vi "initializePIP.vi"(8 "error in (no error)":errorcluster) -> (0 "error out":errorcluster, 2 "Initialize Test":string, 3 "Config and Fixture Setup":string)   [LabVIEW 2018]
uses:
  Global_1259.vi
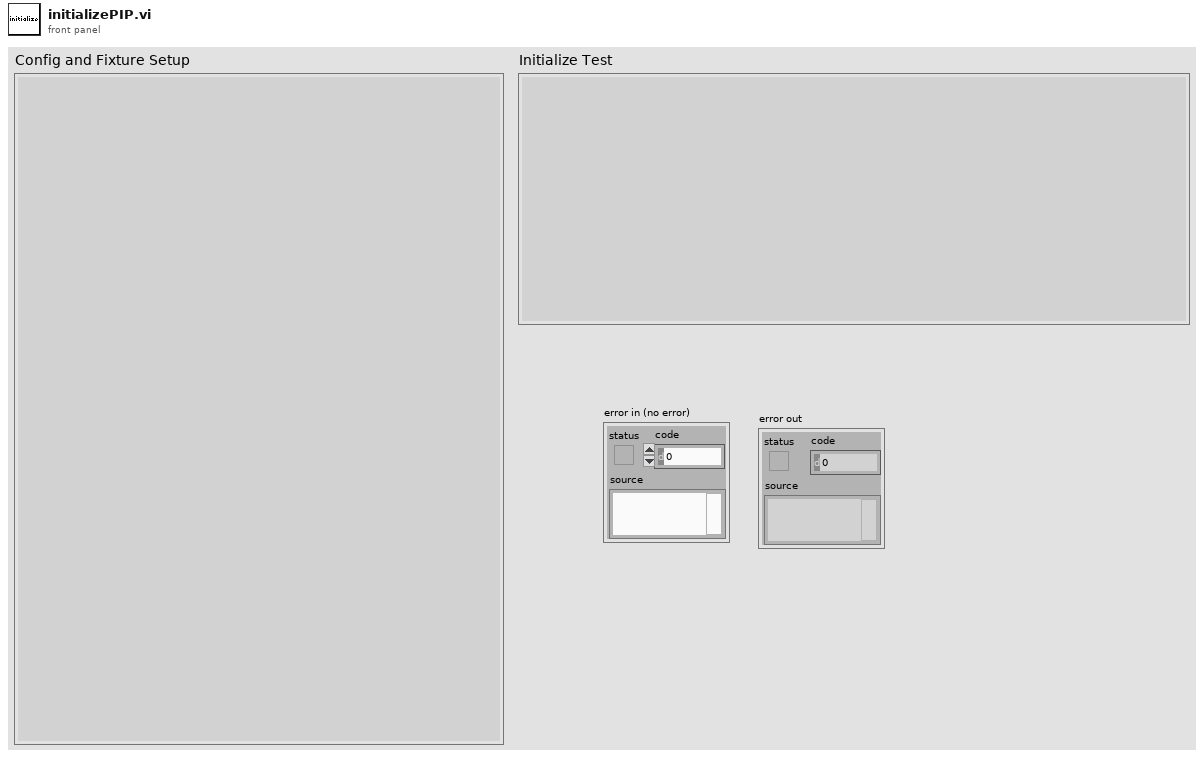
[diagram p1: front panel]
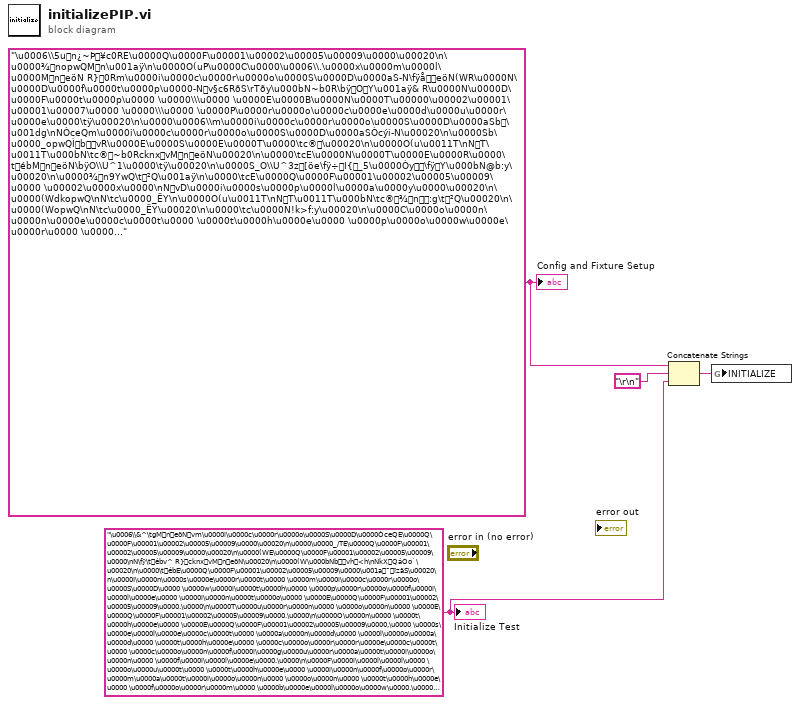
[diagram p0: block diagram]
diagram:
  w4 = "\u0006\\5un¿~Þ¥c0RE\u0000Q\u0000F\u00001\u00002\u00005\u00009\u0000\u00020\n\u0000¾nopwQMn\u001aÿ\n\u0000O(uP\u0000C\u0000\u0006\\.\u0000x\u0000m\u0000l\u0000MneöN R}0Rm\u0000i\u0000c\u0000r\u0000o\u0000S\u0000D\u0000aS-N\fÿåeöN(WR\u0000N\u0000D\u0000f\u0000t\u0000p\u0000-Nv§c6RðS\rTðy\u000bN~b0R\bÿOY\u001aÿ& R\u0000N\u0000D\u0000F\u0000t\u0000p\u0000 \u0000\\\u0000 \u0000E\u0000B\u0000N\u0000T\u00000\u00002\u00001\u00001\u00007\u0000 \u0000\\\u0000 \u0000P\u0000r\u0000o\u0000c\u0000e\u0000d\u0000u\u0000r\u0000e\u0000\tÿ\u00020\n\u0000\u0006\\m\u0000i\u0000c\u0000r\u0000o\u0000S\u0000D\u0000aSb\u001dg\nNÒceQm\u0000i\u0000c\u0000r\u0000o\u0000S\u0000D\u0000aSÒcýi-N\u00020\n\u0000Sb\u0000_opwQÌbvR\u0000E\u0000S\u0000E\u0000T\u0000\tc®\u00020\n\u0000O(u\u0011T\nNT\u0011T\u000bN\tc®~b0RcknxvMneöN\u00020\n\u0000\tcE\u0000N\u0000T\u0000E\u0000R\u0000\tébMneöN\bÿO\\U^1\u0000\tÿ\u00020\n\u0000S_O\\U^3z[öe\fÿ÷I{_5\u0000Òy\fÿY\u000bN@b:y\u00020\n\u0000¾n9YwQ\t²Q\u001aÿ\n\u0000\tcE\u0000Q\u0000F\u00001\u00002\u00005\u00009\u0000 \u00002\u0000x\u0000\nNvD\u0000i\u0000s\u0000p\u0000l\u0000a\u0000y\u0000\u00020\n\u0000(WdkopwQ\nN\tc\u0000_ËY\n\u0000O(u\u0011T\nNT\u0011T\u000bN\tc®¾n:g\t²Q\u00020\n\u0000(WopwQ\nN\tc\u0000_ËY\u00020\n\u0000\tc\u0000N!k>f:y\u00020\n\u0000C\u0000o\u0000n\u0000n\u0000e\u0000c\u0000t\u0000 \u0000t\u0000h\u0000e\u0000 \u0000p\u0000o\u0000w\u0000e\u0000r\u0000 \u0000..."
  w2 = "\u0006\\&^\tgMneöNvm\u0000i\u0000c\u0000r\u0000o\u0000S\u0000D\u0000ÒceQE\u0000Q\u0000F\u00001\u00002\u00005\u00009\u0000\u00020\n\u0000\u0000_/TE\u0000Q\u0000F\u00001\u00002\u00005\u00009\u0000\u00020\n\u0000(WE\u0000Q\u0000F\u00001\u00002\u00005\u00009\u0000\nN\fÿ\tébv^ R}cknxvMneöN\u00020\n\u0000(W\u000bNbvh<h\nNkXQáOo`\u00020\n\u0000\tébE\u0000Q\u0000F\u00001\u00002\u00005\u00009\u0000\u001a¯ïzãS\u00020\n\u0000I\u0000n\u0000s\u0000e\u0000r\u0000t\u0000 \u0000m\u0000i\u0000c\u0000r\u0000o\u0000S\u0000D\u0000 \u0000w\u0000i\u0000t\u0000h\u0000 \u0000p\u0000r\u0000o\u0000f\u0000i\u0000l\u0000e\u0000 \u0000i\u0000n\u0000t\u0000o\u0000 \u0000E\u0000Q\u0000F\u00001\u00002\u00005\u00009\u0000.\u0000\n\u0000T\u0000u\u0000r\u0000n\u0000 \u0000o\u0000n\u0000 \u0000E\u0000Q\u0000F\u00001\u00002\u00005\u00009\u0000.\u0000\n\u0000O\u0000n\u0000 \u0000t\u0000h\u0000e\u0000 \u0000E\u0000Q\u0000F\u00001\u00002\u00005\u00009\u0000,\u0000 \u0000s\u0000e\u0000l\u0000e\u0000c\u0000t\u0000 \u0000a\u0000n\u0000d\u0000 \u0000l\u0000o\u0000a\u0000d\u0000 \u0000t\u0000h\u0000e\u0000 \u0000c\u0000o\u0000r\u0000r\u0000e\u0000c\u0000t\u0000 \u0000c\u0000o\u0000n\u0000f\u0000i\u0000g\u0000u\u0000r\u0000a\u0000t\u0000i\u0000o\u0000n\u0000 \u0000f\u0000i\u0000l\u0000e\u0000.\u0000\n\u0000F\u0000i\u0000l\u0000l\u0000 \u0000o\u0000u\u0000t\u0000 \u0000t\u0000h\u0000e\u0000 \u0000i\u0000n\u0000f\u0000o\u0000r\u0000m\u0000a\u0000t\u0000i\u0000o\u0000n\u0000 \u0000o\u0000n\u0000 \u0000t\u0000h\u0000e\u0000 \u0000f\u0000o\u0000r\u0000m\u0000 \u0000b\u0000e\u0000l\u0000o\u0000w\u0000.\u0000\n\u0000S\u0000e\u0000l\u0000e\u0000c\u0000t\u0000 \u0000t\u0000h\u0000e\u0000 \u0000E\u0000Q\u0000F\u00001\u00002\u00005\u00009\u0000 \u0000c\u0000o\u0000m\u0000m\u0000u\u0000n\u0000i\u0000c\u0000a\u0000t\u0000i\u0000o\u0000n\u0000 \u0000p\u0000o\u0000r\u0000t\u0000.\u0000"
  n1 = Concatenate Strings(w4, "\r\n", w2) -> (w1:string)
  n2 = global write "Global_1259.vi" "INITIALIZE"(w1) -> ()
  "Initialize Test" <- w2
  "Config and Fixture Setup" <- w4
